vi "JAX.vi"(0 "System no.":i32=1 min=1 max=4 step=1, 1 "JoystickID":i32, 2 "Joystick axis":i32, 3 "Axes to set":string[](array[string]), 5 "error in":errorcluster) -> (19 "error out":errorcluster)   [LabVIEW 2020]
doc: "Defines which axes to control with an axis of a joystick connected to the controller. If Axes to set is an empty array, the current settings are cleared and no axes are controlled. Joystick control is enabled or disabled with JON.vi. Settings will not influence Joystick_Operation_Sample_Program.vi which works with a joystick connected to the host computer.\n\nE-709: Only supported if E-709 is used inside C-867K012/K013."
uses:
  <vilib>/Utility/error.llb/whitespace.ctl
panel:
  # "Defines  which axes to control with an axis of a joystick connected\nto the controller. If Axes to set is an empty array, the current \nsettings are cleared and no axes are controlled."
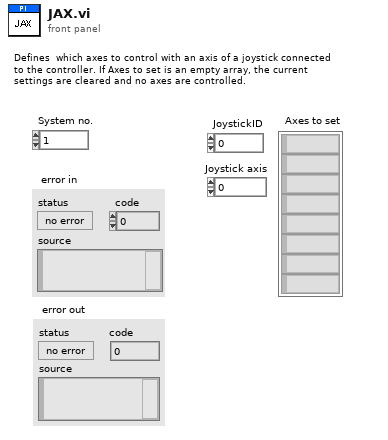
[diagram p1: front panel]
types:
  T1 = typedef "whitespace.ctl" = u16
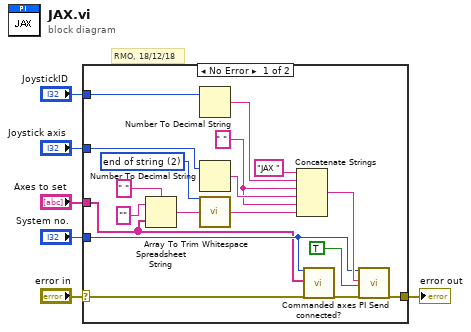
[diagram p0: block diagram]
diagram:
  # "RMO, 18/12/18"
  n1 = case shown="No Error" "error in" {
    selector: "error in" -> [w7 w25]
    tunnel: "Joystick axis" -> [w19 _]
    tunnel: "JoystickID" -> [w20 _]
    tunnel: "System no." -> [w10 _]
    tunnel: [w24 w25] -> w5
    tunnel: "Axes to set" -> [w9 _]
    frame No Error {
      w12 = T1 2 items=["both", "start of string", "end of string"] ("location (both)")
      w16 = " " ("string")
      n2 = Array To Spreadsheet String(delimiter (Tab)=" ", array=w9, 3:"" ("format string")) -> (spreadsheet string=w13:string)
      n3 = Number To Decimal String(number=w20) -> (decimal integer string=w18:string)  [unwired: 1 out]
      n4 = Number To Decimal String(number=w19) -> (decimal integer string=w17:string)  [unwired: 1 out]
      n5 = call <vilib>:"Trim Whitespace.vi"("string"=w13, "location (both)"=w12) -> ("trimmed string"=w11:string)
      n6 = Concatenate Strings("JAX ", w18, w16, w17, w16, w11) -> (w21:string)
      n7 = call "Commanded axes connected?.vi"("System no."=w10, "Commanded axes"=w9, "error in"=w7) -> ("error out"=w8:errorcluster)  [unwired: 16 out]
      n8 = call "PI Send.vi"("System no."=w10, "String to send"=w21, "Attach termination char.?"=TRUE ("Attach Linefeed?"), "error in"=w8) -> ("error out"=w24:errorcluster)  [unwired: 2 in, 13 out]
    }
    frame Error {
    }
  }
  "error out" <- w5
